vi "Insert Cell.vi"(6 "Reinsert?":bool, 8 "error in (no error)":errorcluster, 10 "Schedule Cell":refnum<class "Schedule Cell.lvclass">, 11 "Schedule in":refnum<class "Schedule.lvclass">) -> (0 "error out":errorcluster, 3 "Schedule out":refnum<class "Schedule.lvclass">)   [LabVIEW 2020, in "Run Utilities.lvlib" / "Schedule.lvclass"]
uses:
  Schedule.lvclass
  Cell/Schedule Cell.lvclass
  Schedule.lvclass/Schedule.ctl
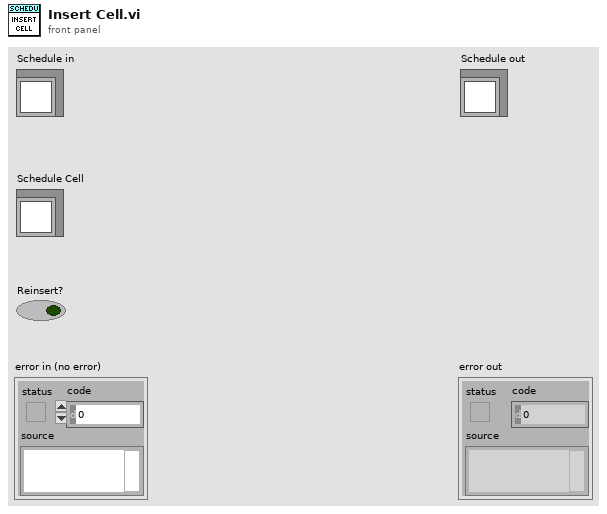
[diagram p1: front panel]
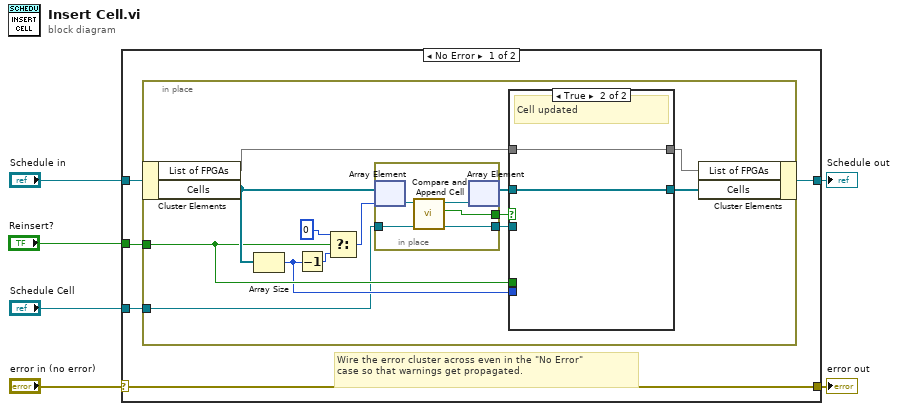
[diagram p0: block diagram]
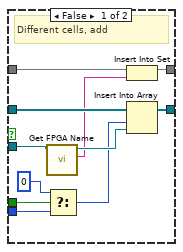
[diagram p2: hidden frame]
diagram:
  n1 = case shown="No Error" "error in (no error)" {
    selector: "error in (no error)" -> [w11 w44]
    tunnel: [w11 w44] -> w5
    tunnel: [w9 w43] -> w3
    tunnel: "Schedule in" -> [w10 w43]
    tunnel: "Schedule Cell" -> [w8 _]
    tunnel: "Reinsert?" -> [w7 _]
    frame No Error {
      # "Wire the error cluster across even in the \"No Error\"\ncase so that warnings get propagated."
      n2 = in-place {
        in-place-border: w8 -> [w14]
        in-place-border: w7 -> [w16]
        n3 = in-place-cluster #1(w10) -> ("List of FPGAs"=w13:set{string}, "Cells"=w18:refnum<class "Schedule Cell.lvclass">[])
        n4 = Array Size(array=w18) -> (size(s)=w15:i32)
        n5 = Decrement(x=w15) -> (x-1=w20:i32)
        n6 = Select(t=0, s=w16, f=w20) -> (s? t:f=w17:i32)
        n7 = in-place {
          in-place-border: w14 -> [w27]
          in-place-border: [w26] -> w22
          in-place-border: [w25] -> w21
          n8 = in-place-array #2(w18, w17) -> (w29:refnum<class "Schedule Cell.lvclass">)
          n9 = call-dynamic "Compare and Append Cell.vi"("Schedule Cell B in"=w27, "Schedule Cell A in"=w29) -> ("Schedule Cell B out"=w26:refnum<class "Schedule Cell.lvclass">, "Cell Updated"=w25:bool, "Schedule Cell A out"=w28:refnum<class "Schedule Cell.lvclass">)  [unwired: 7 in]
          n10 = in-place-array #2(w28) -> (w23:refnum<class "Schedule Cell.lvclass">[])  [unwired: 1 out]
        }
        n11 = case shown="True" w21 {
          tunnel: w23 -> [w40 w42]
          tunnel: w22 -> [w33 _]
          tunnel: [w39 w42] -> w24
          tunnel: w16 -> [w38 _]
          tunnel: w15 -> [w37 _]
          tunnel: w13 -> [w35 w41]
          tunnel: [w34 w41] -> w12
          frame False {
            # "Different cells, add"
            n12 = call-dynamic "Get FPGA Name.vi"("Schedule Cell in"=w33) -> ("FPGA Name"=w31:string, "Schedule Cell out"=w32:refnum<class "Schedule Cell.lvclass">)  [unwired: 8 in, 1 out]
            n13 = Select(t=0, s=w38, f=w37) -> (s? t:f=w30:i32)
            n14 = Insert Into Set(10:w31, 11:w35) -> (3:w34:set{string})  [unwired: 1 out]
            n15 = Insert Into Array(array=w40, index=w30, new element=w32) -> (w39:refnum<class "Schedule Cell.lvclass">[])
          }
          frame True {
            # "Cell updated"
          }
        }
        n16 = in-place-cluster #1("List of FPGAs"=w12, "Cells"=w24) -> (w9:refnum<class "Schedule.lvclass">)
      }
    }
    frame Error {
    }
  }
  "error out" <- w5
  "Schedule out" <- w3
